vi "nominal channel search.vi"(0 "client":i32, 1 "out_list":i32, 5 "data_source_rid":string, 7 "substring":string, 9 "data_type":i32, 11 "error in (no error)":errorcluster, 12 "out_count":u32) -> (3 "out_list out":i32, 4 "function return":i32, 14 "out_count out":u32, 15 "error out":errorcluster)   [LabVIEW 2020, in "client.lvlib"]
doc: "int32_t nominal_channel_search(int32_t client,\n const char *data_source_rid,\n const char *substring,\n int32_t data_type,\n int32_t *out_list,\n uint32_t *out_count);"
uses:
  client.lvlib
  nominalClient_64.dll
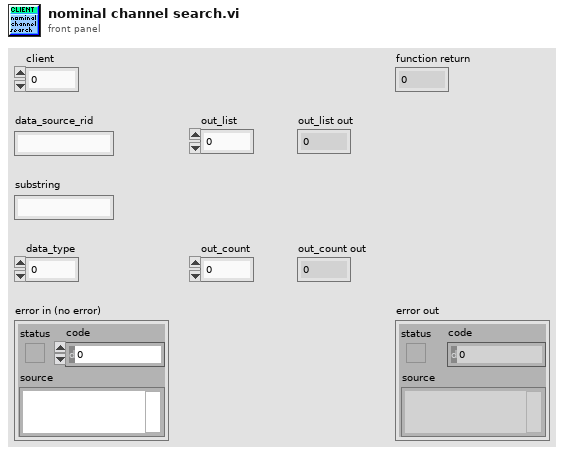
[diagram p1: front panel]
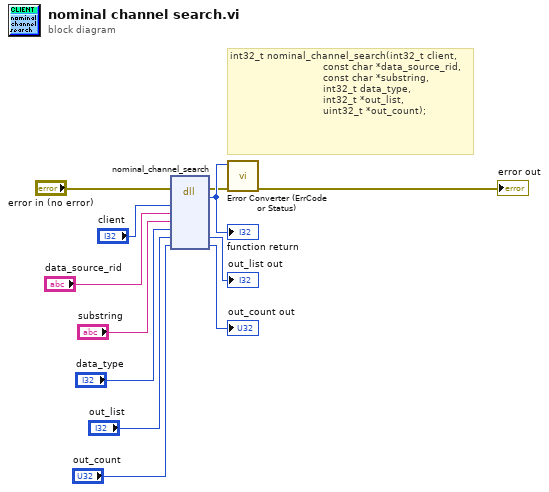
[diagram p0: block diagram]
diagram:
  # "int32_t nominal_channel_search(int32_t client,\n                               const char *data_source_rid,\n                               const char *substring,\n                               int32_t data_type,\n                               int32_t *out_list,\n                               uint32_t *out_count);"
  n1 = dll-call lib="C:/code/labview-client-rs/lv_src/client/nominalClient_*.*" fn="nominal_channel_search"(error in="error in (no error)", "client"="client", "data_source_rid"="data_source_rid", "substring"="substring", "data_type"="data_type", "out_list"="out_list", "out_count"="out_count") -> (error out=w2:errorcluster, w12:i32, "out_list"=→"out_list out":i32, "out_count"=→"out_count out":u32)  [unwired: 6 in, 1 out]
  "function return" <- w12
  n2 = call "Error Converter (ErrCode or Status).vi"("error in (no error)"=w2, "error code"=w12) -> ("error out"=→"error out":errorcluster)  [unwired: 9 in]
